vi "Launch Timer.vi"(6 "Log time":T1, 7 "Timer name":string="Timer", 8 "error in (no error)":errorcluster, 10 "Timer period":u32=1000, 11 "Mag Lab Measure Controller in":refnum<class "Mag Lab Measure Controller.lvclass">) -> (0 "error out":errorcluster, 3 "Mag Lab Measure Controller out":refnum<class "Mag Lab Measure Controller.lvclass">)   [LabVIEW 2015, in "Mag Lab Measure Controller.lvclass"]
uses:
  Mag Lab Measure Controller.lvclass
  Measurement Timer/Log time.ctl
  Measurement Timer/Measurement Timer.lvclass
  Mag Lab Measure Controller.lvclass/Mag Lab Measure Controller.ctl
  <vilib>/ActorFramework/Message Enqueuer/Message Enqueuer.lvclass/Message Enqueuer.ctl
  Measurement Timer/Measurement Timer.lvclass/Measurement Timer.ctl
  <vilib>/ActorFramework/Message Enqueuer/Enqueue.vi
  <vilib>/ActorFramework/Message Priority Queue/Priority Enqueue.vi
  <vilib>/ActorFramework/Message Enqueuer/Message Enqueuer.lvclass
  <vilib>/ActorFramework/Stop Msg/Stop Msg.lvclass
  Mag Lab Error Handler/Mag Lab Error Handler.lvclass
  Mag Lab Measure Base/Mag Lab Measure Base.lvclass
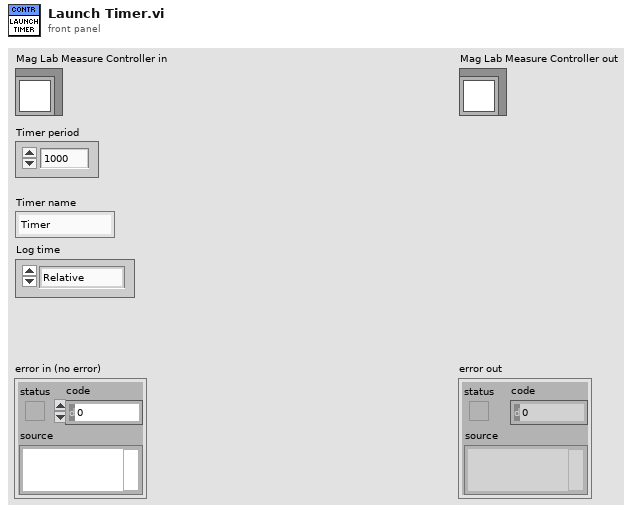
[diagram p1: front panel]
types:
  T1 = typedef "Log time.ctl" = enum16{"Relative", "Absolute", "Do not log"}
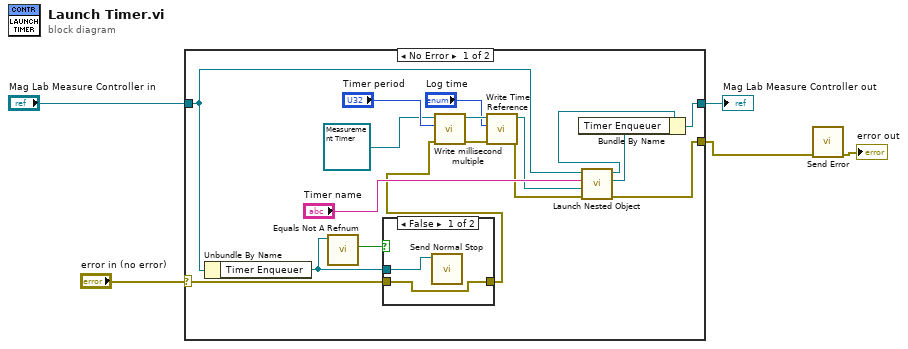
[diagram p0: block diagram]
diagram:
  n1 = case shown="No Error" "error in (no error)" {
    selector: "error in (no error)" -> [w20 w27]
    tunnel: [w8 w27] -> w2
    tunnel: [w21 w26] -> w3
    tunnel: "Mag Lab Measure Controller in" -> [w14 w26]
    frame No Error {
      n2 = Unbundle By Name(w14) -> ("Timer Enqueuer"=w15:refnum<class "Message Enqueuer.lvclass">)
      n3 = call <vilib>:"Equals Not A Refnum.vi"("Message Enqueuer"=w15) -> ("Not a refnum?"=w19:bool)  [unwired: 10 in]
      n4 = case shown="False" w19 {
        tunnel: w20 -> [w23 w25]
        tunnel: [w23 w25] -> w7
        tunnel: w15 -> [w24 _]
        frame False {
          n5 = call <vilib>:"Send Normal Stop.vi"("Message Enqueuer"=w24) -> ()  [unwired: 10 in, 1 out]
        }
        frame True {
        }
      }
      n6 = call "Write millisecond multiple.vi"("error in (no error)"=w7, "millisecond multiple"="Timer period", "Measurement Timer in"=refnum<class "Measurement Timer.lvclass"> refnum ("Measurement Timer.lvclass")) -> ("error out"=w16:errorcluster, "Measurement Timer out"=w18:refnum<class "Measurement Timer.lvclass">)  [unwired: 7 in]
      n7 = call "Write Time Reference.vi"("error in (no error)"=w16, "Report time as result"="Log time", "Measurement Timer in"=w18) -> ("error out"=w9:errorcluster, "Measurement Timer out"=w12:refnum<class "Measurement Timer.lvclass">)  [unwired: 7 in]
      n8 = call "Launch Nested Object.vi"("error in (no error)"=w9, "Object"=w12, "name"="Timer name", "Mag Lab Measure Base in"=w14) -> ("error out"=w8:errorcluster, "Caller-To-Actor Enqueuer"=w10:refnum<class "Message Enqueuer.lvclass">, "Mag Lab Measure Base out"=w11:refnum<class "Mag Lab Measure Controller.lvclass">)  [unwired: 5 in]
      n9 = Bundle By Name(cluster=w11, "Timer Enqueuer"=w10) -> (w21:refnum<class "Mag Lab Measure Controller.lvclass">)
    }
    frame Error {
    }
  }
  "Mag Lab Measure Controller out" <- w3
  n10 = call "Send Error.vi"("error in (no error)"=w2) -> ("error out"=→"error out":errorcluster)  [unwired: 9 in, 1 out]
